vi "E3640A GP Commands SA.vi"() -> ()   [LabVIEW 2009]
uses:
  <vilib>/Instr/_visa.llb/VISA Configure Serial Port (Instr).vi
panel:
  out "Num Resp":dbl
  in  "Command":string(combo)
  out "Bytes at port":u8
  out "Bytes Read":u8
  out "Response":string
  in  "Serial Configuration":T1={"Baud Rate"=9600, "Parity"=0, "Data Bits"=8, "Stop Bits"=20, "Flow Control"=0} {"Flow Control" items=["None", "XON/XOFF", "RTS/CTS", "XON/XOFF & RTS/CTS", "DTR/DSR", "XON/XOFF & DTR/DSR"]; "Stop Bits" items=["1.0"=10, "1.5"=15, "2.0"=20]; "Data Bits" items=["7"=7, "8"=8]; "Parity" items=["None", "Odd", "Even", "Mark", "Space"]; "Baud Rate" items=["300"=300, "600"=600, "1200"=1200, "2400"=2400, "4800"=4800, "9600"=9600, "19200"=19200]}
  in  "VISA session":refnum<visa-resource-name>="COM4"
  out "error out":errorcluster
  in  "error in (no error)":errorcluster
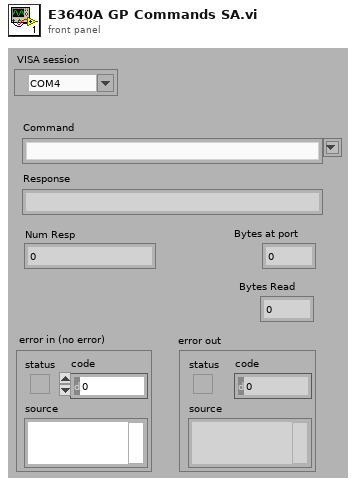
[diagram p1: front panel]
types:
  T1 = cluster{"Baud Rate":u32, "Parity":u16, "Data Bits":u16, "Stop Bits":u16, "Flow Control":u16}
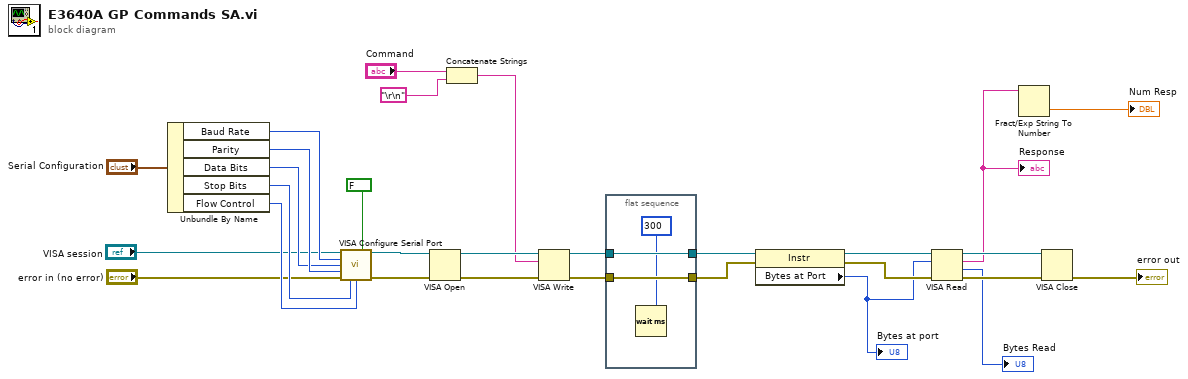
[diagram p0: block diagram]
diagram:
  n1 = Unbundle By Name("Serial Configuration") -> ("Baud Rate"=w28:u32, "Parity"=w27:u16, "Data Bits"=w26:u16, "Stop Bits"=w25:u16, "Flow Control"=w24:u16)
  n2 = call-poly "VISA Configure Serial Port"("VISA resource name"="VISA session", "Enable Termination\nChar (T)"=FALSE, "baud rate (9600)"=w28, "data bits (8)"=w26, "parity (0:none)"=w27, "error in (no error)"="error in (no error)", "stop bits (10: 1 bit)"=w25, "flow control (0:none)"=w24) -> ("VISA resource name out"=w20:refnum<visa-resource-name>, "error out"=w19:errorcluster)  [unwired: 6 in]
  n3 = VISA Open(error in (no error)=w19, VISA resource name=w20) -> (VISA resource name=w17:refnum<visa-resource-name>, error out=w18:errorcluster)  [unwired: 3 in]
  n4 = Concatenate Strings("Command", "\r\n") -> (w15:string)
  n5 = VISA Write(VISA resource name=w17, write buffer=w15, error in (no error)=w18) -> (VISA resource name out=w7:refnum<visa-resource-name>, error out=w6:errorcluster)  [unwired: 1 out]
  n6 = flat-sequence {
    tunnel: [w32] -> w4
    tunnel: w7 -> [w32]
    tunnel: [w31] -> w5
    tunnel: w6 -> [w31]
    frame #0 {
      n7 = Wait (ms)(milliseconds to wait=300) -> ()  [unwired: 1 out]
    }
  }
  n8 = property class="Instr"(reference=w4, error in=w5) -> (reference out=w10:refnum<visa-resource-name>, error out=w9:errorcluster, "Bytes at Port"=w8:u32)
  "Bytes at port" <- w8
  n9 = VISA Read(VISA resource name=w10, byte count=w8, error in (no error)=w9) -> (VISA resource name out=w13:refnum<visa-resource-name>, read buffer=w2:string, return count=→"Bytes Read":u32, error out=w12:errorcluster)
  "Response" <- w2
  n10 = Fract/Exp String To Number(string=w2) -> (number=→"Num Resp":dbl)  [unwired: 3 in, 1 out]
  n11 = VISA Close(VISA resource name=w13, error in (no error)=w12) -> (error out=→"error out":errorcluster)
